vi "run_experiment_multi_mix.vi"(4 "Sync Camera Acquisition":bool, 5 "Log File Name":path, 7 "Pressure Sequence":dbl[][](array[numeric]), 8 "Valve Sequence Data":T2(array[cluster]), 9 "mixture sequence array":string[](array[string]), 10 "Time Sequence":dbl[](array[numeric]), 11 "MFCS_EZ":T3) -> (0 "Aborted?":bool, 3 "Flow Data Out":T1)   [LabVIEW 2016]
uses:
  <userlib>/Fluigent/Fluigent MFCS/FluigentMFCS_Full.llb/_EZmfcsRefNum.ctl
  <userlib>/Fluigent/Fluigent MFCS/FluigentMFCS_Full.llb/_EZmfcsEnum.ctl
  <userlib>/Fluigent/Fluigent MFCS/FluigentMFCS_Full.llb/MFCS_EZ Write Channel Pressure.vi
  Globals/PressuresGlobal.vi
panel:
  out "Log File Name":path
  in  "stop":bool
  out "Step Time":u8(slide) scale=0.0..100.0
  out "Current State":string
  out "Remaining Time":dbl
  out "Experiment Progress":u8(slide) scale=0.0..100.0
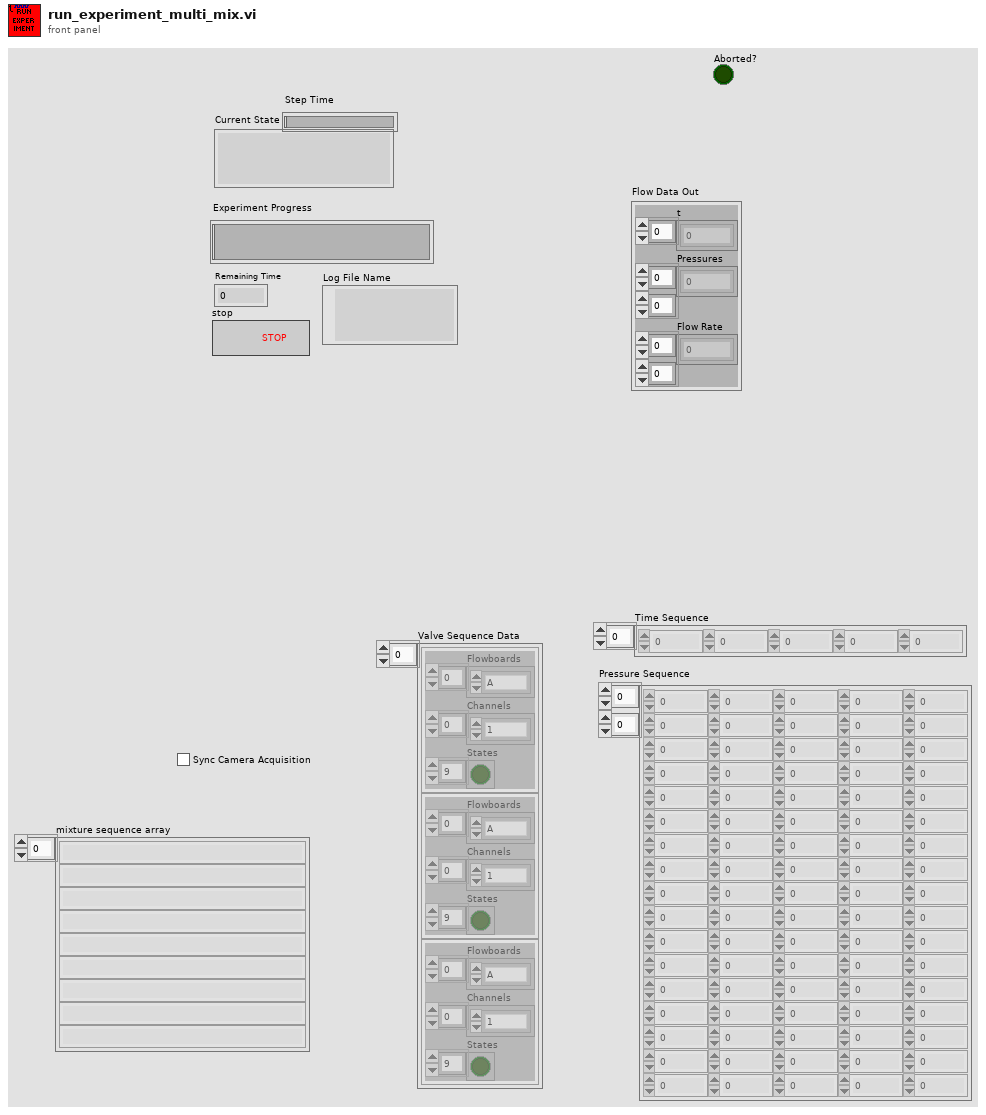
[diagram p1: front panel]
types:
  T1 = cluster{"t":dbl[], "Pressures":dbl[][], "Flow Rate":dbl[][]}
  T2 = cluster{"Flowboards":enum16{"A", "B", "C"}[], "Channels":enum16{"1", "2", "3", "4", "5", "6", "7", "8"}[], "States":bool[]}[]
  T3 = typedef "_EZmfcsRefNum.ctl" = refnum<k1>
  T4 = enum16{"Release", "Create", "Send", "Wait", "Cancel"}
  T5 = cluster{"Flowboards":enum16{"A", "B", "C"}[], "Channels":enum16{"1", "2", "3", "4", "5", "6", "7", "8"}[], "States":bool[]}
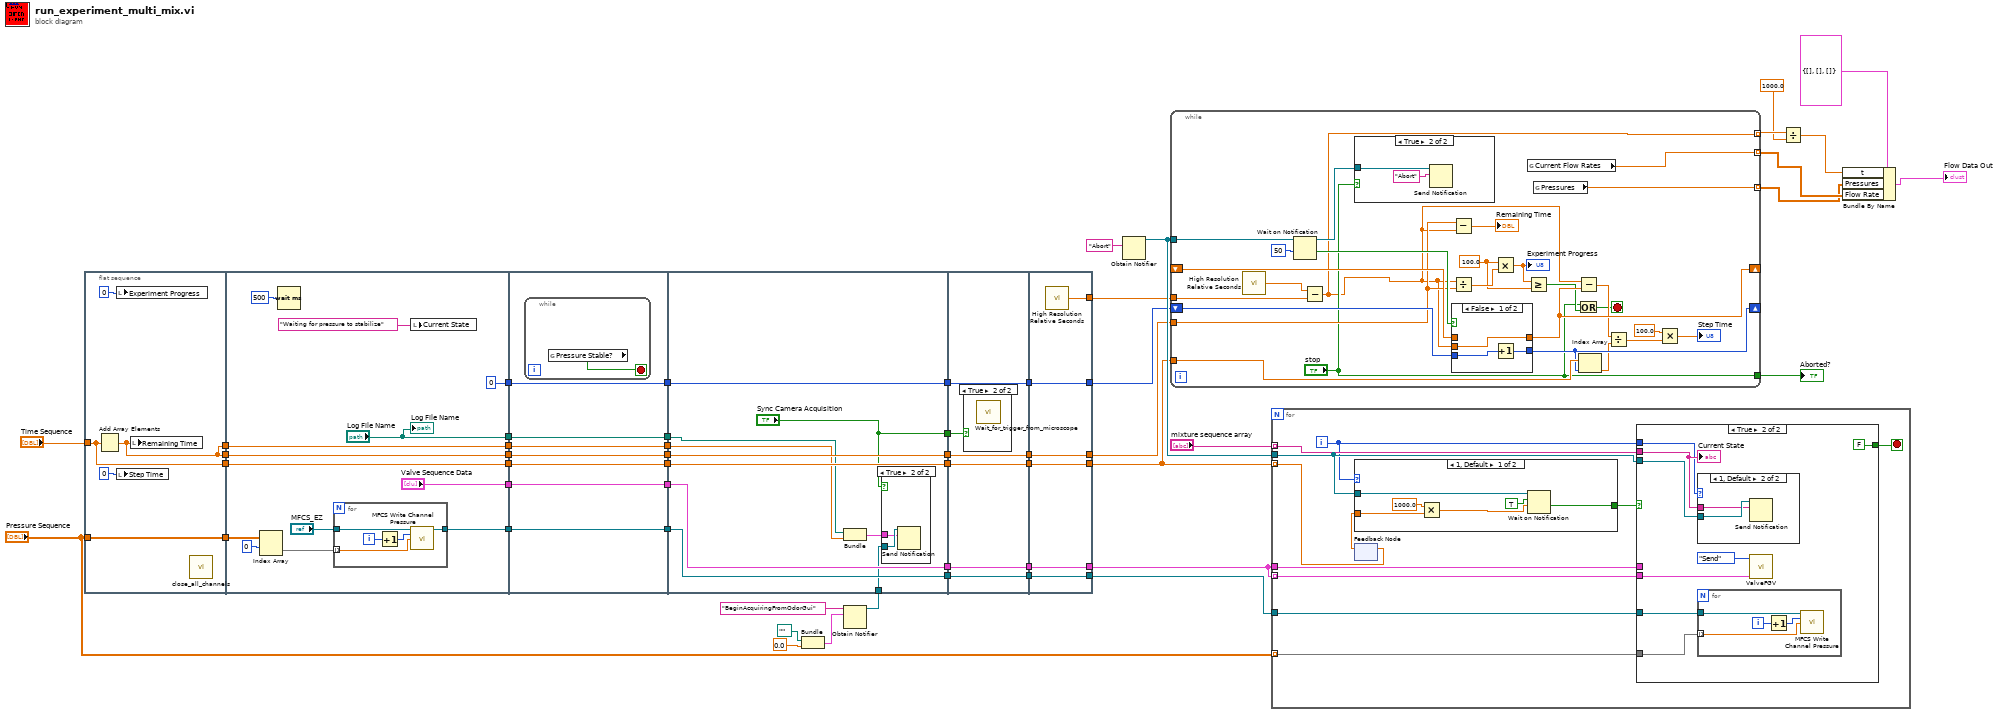
[diagram p0: block diagram]
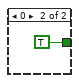
[diagram p6: hidden frame]
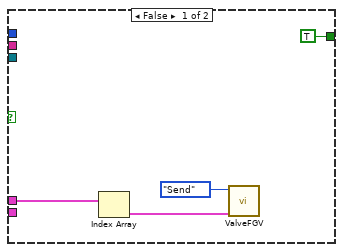
[diagram p7: hidden frame]
diagram:
  n1 = flat-sequence {
    tunnel: "Pressure Sequence" -> [w58]
    tunnel: [w58] -> w48
    tunnel: "Time Sequence" -> [w55]
    tunnel: [w55] -> w41
    tunnel: [w54] -> w40
    tunnel: [w54] -> w21
    tunnel: w48 -> [w61]
    tunnel: [w67] -> w38
    tunnel: ["Valve Sequence Data"] -> w37
    tunnel: [0] -> w36
    tunnel: [w65] -> w35
    tunnel: [w64] -> w34
    tunnel: w41 -> [w65]
    tunnel: w40 -> [w64]
    tunnel: [w63] -> w22
    tunnel: w21 -> [w63]
    tunnel: ["Log File Name"] -> w8
    tunnel: w38 -> [w83]
    tunnel: [w83] -> w29
    tunnel: w37 -> [w82]
    tunnel: [w82] -> w28
    tunnel: w36 -> [w81]
    tunnel: [w81] -> w27
    tunnel: w35 -> [w80]
    tunnel: [w80] -> w26
    tunnel: w34 -> [w79]
    tunnel: [w79] -> w25
    tunnel: [w78] -> w23
    tunnel: w22 -> [w78]
    tunnel: [w77] -> w9
    tunnel: w8 -> [w77]
    tunnel: w29 -> [w94]
    tunnel: [w94] -> w20
    tunnel: w28 -> [w93]
    tunnel: [w93] -> w18
    tunnel: w27 -> [w92]
    tunnel: [w92] -> w16
    tunnel: w26 -> [w91]
    tunnel: [w91] -> w14
    tunnel: w25 -> [w90]
    tunnel: [w90] -> w12
    tunnel: w24 -> [w88]
    tunnel: w23 -> [w87]
    tunnel: ["Sync Camera Acquisition"] -> w10
    tunnel: w9 -> [w85]
    tunnel: w20 -> [w102]
    tunnel: [w102] -> w19
    tunnel: w18 -> [w101]
    tunnel: [w101] -> w17
    tunnel: w16 -> [w100]
    tunnel: [w100] -> w15
    tunnel: w14 -> [w99]
    tunnel: [w99] -> w13
    tunnel: w12 -> [w98]
    tunnel: [w98] -> w11
    tunnel: w10 -> [w97]
    tunnel: [w104] -> w45
    tunnel: [w105] -> w46
    tunnel: [w106] -> w47
    tunnel: [w107] -> w43
    tunnel: [w108] -> w49
    tunnel: w19 -> [w108]
    tunnel: w17 -> [w107]
    tunnel: w15 -> [w106]
    tunnel: w13 -> [w105]
    tunnel: w11 -> [w104]
    tunnel: [w103] -> w44
    frame #0 {
      n2 = Add Array Elements(numeric array=w55) -> (sum=w54:dbl)
      n3 = local write "Experiment Progress"(u8 0 ("Experiment Progress")) -> ()
      n4 = local write "Step Time"(u8 0 ("Step Time")) -> ()
      n5 = local write "Remaining Time"(w54) -> ()
      n6 = call "close_all_channels.vi"() -> ()  [unwired: 12 in]
    }
    frame #1 {
      n7 = Index Array(array=w61, index (row)=0) -> (element=w59:dbl[])  [unwired: 1 in]
      n8 = Wait (ms)(milliseconds to wait=u32 500) -> ()  [unwired: 1 out]
      n9 = for {
        tunnel: "MFCS_EZ" -> [w76]
        tunnel: w59 -> [w75] mode=indexing
        tunnel: [w74] -> w67
        i -> [w73]
        n10 = Increment(x=w73) -> (x+1=w72:i32)
        n11 = call-poly <userlib>:"MFCS Write Channel Pressure.vi"("MFCS_EZ"=w76, "Channel Number (default=1)"=w72, "Pressure (mBar)"=w75) -> ("MFCS_EZ out"=w74:T3)  [unwired: 11 in, 1 out]
      }
      n12 = local write "Current State"("Waiting for pressure to stabilize" ("Current State")) -> ()
      "Log File Name" <- "Log File Name"
    }
    frame #2 {
      n13 = while {
        stop <- w84 stop-if-true
        n14 = global read "PressuresGlobal.vi" "Pressure Stable?"() -> (w84:bool)
      }
    }
    frame #3 {
      n15 = Bundle("Log File Name"=w85, "Start Water"=w87) -> (w89:cluster{"Log File Name":path, "Start Water":dbl})  [unwired: 1 in]
      n16 = case shown="True" "Sync Camera Acquisition" {
        tunnel: w88 -> [_ w96]
        tunnel: w89 -> [_ w95]
        frame False {
        }
        frame True {
          n17 = Send Notification(notification=w95, notifier=w96) -> ()  [unwired: 1 in, 2 out]
        }
      }
    }
    frame #4 {
      n18 = case shown="True" w97 {
        frame False {
        }
        frame True {
          n19 = call "Wait_for_trigger_from_microscope.vi"() -> ()  [unwired: 12 in]
        }
      }
    }
    frame #5 {
      n20 = call <vilib>:"High Resolution Relative Seconds.vi"() -> ("relative seconds"=w103:dbl)
    }
  }
  n21 = Bundle("Log File Name"=path "", 0.0) -> (w31:cluster{"Log File Name":path, dbl})  [unwired: 1 in]
  n22 = Obtain Notifier(name (unnamed)="BeginAcquiringFromOdorGui", notification data type=w31) -> (notifier out=w24:refnum<notifier>)  [unwired: 2 in, 2 out]
  n23 = Obtain Notifier(notification data type="Abort" ("notification")) -> (notifier out=w53:refnum<notifier>)  [unwired: 3 in, 2 out]
  n24 = while {
    tunnel: w53 -> [w132]
    tunnel: w45 -> [w123]
    tunnel: w44 -> [w135]
    tunnel: w46 -> [w128]
    shift-right: [w119] -> _
    shift-left: _ -> [w129]
    shift-right: [w126] -> _
    shift-left: w47 -> [w127]
    tunnel: ["stop"] -> w39
    tunnel: [w112] -> w3 mode=indexing
    tunnel: [w109] -> w7 mode=indexing
    tunnel: [w110] -> w2 mode=indexing
    stop <- w114 stop-if-true
    w116 = 100.0 ("x")
    n25 = call <vilib>:"High Resolution Relative Seconds.vi"() -> ("relative seconds"=w111:dbl)
    n26 = Wait on Notification(notifier=w132, timeout in ms (-1)=50) -> (notifier out=w124:refnum<notifier>, timed out?=w130:bool)  [unwired: 2 in, 2 out]
    n27 = Subtract(x=w111, y=w135) -> (x-y=w109:dbl)
    n28 = case shown="True" "stop" {
      tunnel: w124 -> [_ w137]
      frame False {
      }
      frame True {
        n29 = Send Notification(notification="Abort", notifier=w137) -> ()  [unwired: 1 in, 2 out]
      }
    }
    n30 = Subtract(x=w123, y=w109) -> (x-y=→"Remaining Time":dbl)
    n31 = Divide(x=w109, y=w123) -> (x/y=w133:dbl)
    n32 = case shown="False" w130 {
      tunnel: w109 -> [w140 _]
      tunnel: [w140 w142] -> w119
      tunnel: w129 -> [_ w142]
      tunnel: w127 -> [w139 w141]
      tunnel: [w138 w141] -> w126
      frame False {
        n33 = Increment(x=w139) -> (x+1=w138:i32)
      }
      frame True {
      }
    }
    n34 = Multiply(x=w116, y=w133) -> (x*y=w117:dbl)
    "Experiment Progress" <- w117
    n35 = Greater Or Equal?(x=w117, y=w116) -> (x >= y?=w115:bool)
    n36 = global read "PressuresGlobal.vi" "Current Flow Rates"() -> (w112:dbl[])
    n37 = global read "PressuresGlobal.vi" "Pressures"() -> (w110:dbl[])
    n38 = Subtract(x=w109, y=w119) -> (x-y=w118:dbl)
    n39 = Or(x="stop", y=w115) -> (x .or. y?=w114:bool)
    n40 = Index Array(array=w128, index=w126) -> (element=w125:dbl)
    n41 = Divide(x=w118, y=w125) -> (x/y=w121:dbl)
    n42 = Multiply(x=100.0, y=w121) -> (x*y=→"Step Time":dbl)
  }
  "Aborted?" <- w39
  n43 = for {
    tunnel: w53 -> [w147]
    tunnel: w46 -> [w146] mode=indexing
    tunnel: w43 -> [w152] mode=indexing
    tunnel: "mixture sequence array" -> [w151] mode=indexing
    tunnel: "Pressure Sequence" -> [w150] mode=indexing
    tunnel: w49 -> [w149]
    tunnel: w43 -> [w143]
    i -> [w144]
    stop <- w148 stop-if-true
    n44 = feedback-in #1(w146) -> ()
    n45 = feedback #1() -> (w145:dbl)  [unwired: 1 in]
    n46 = case shown="1, Default" w144 {
      tunnel: w145 -> [w159 _]
      tunnel: [w156 TRUE ("timed out?")] -> w153
      tunnel: w147 -> [w154 _]
      frame 1, Default {
        n47 = Multiply(x=1000.0, y=w159) -> (x*y=w158:dbl)
        n48 = Wait on Notification(notifier=w154, ignore previous (F)=TRUE, timeout in ms (-1)=w158) -> (timed out?=w156:bool)  [unwired: 1 in, 3 out]
      }
      frame 0 {
      }
    }
    n49 = case shown="True" w153 {
      tunnel: w152 -> [_ w169]
      tunnel: w151 -> [_ w167]
      tunnel: w150 -> [_ w171]
      tunnel: w149 -> [_ w172]
      tunnel: w147 -> [_ w168]
      tunnel: [TRUE FALSE] -> w148
      tunnel: w144 -> [_ w165]
      tunnel: w143 -> [w162 _]
      frame False {
        n50 = Index Array(array=w162) -> (element=w161:T5)  [unwired: 1 in]
        n51 = call "ValveFGV.vi"("Valve Data"=w161, "Action"=T4."Send") -> ()  [unwired: 6 in, 4 out]
      }
      frame True {
        n52 = case shown="1, Default" w165 {
          tunnel: w168 -> [_ w174]
          tunnel: w167 -> [_ w173]
          frame 0 {
          }
          frame 1, Default {
            n53 = Send Notification(notification=w173, notifier=w174) -> ()  [unwired: 1 in, 2 out]
          }
        }
        n54 = for {
          tunnel: w172 -> [w178]
          tunnel: w171 -> [w177] mode=indexing
          i -> [w176]
          n55 = Increment(x=w176) -> (x+1=w175:i32)
          n56 = call-poly <userlib>:"MFCS Write Channel Pressure.vi"("MFCS_EZ"=w178, "Channel Number (default=1)"=w175, "Pressure (mBar)"=w177) -> ()  [unwired: 11 in, 2 out]
        }
        n57 = call "ValveFGV.vi"("Valve Data"=w169, "Action"=T4."Send") -> ()  [unwired: 6 in, 4 out]
        "Current State" <- w167
      }
    }
  }
  n58 = Divide(x=w7, y=1000.0) -> (x/y=w4:dbl[])
  n59 = Bundle By Name(cluster=T1 {"t"=[], "Pressures"=[], "Flow Rate"=[]} ("Flow Data Out"), "t"=w4, "Pressures"=w2, "Flow Rate"=w3) -> (→"Flow Data Out":T1)
